vi "Autosort Populate Ring Control.vi"(8 "error in (no error)":errorcluster, 10 "Selected Index":i32, 11 "Ring Refnum":refnum<vi>) -> (0 "error out":errorcluster)   [LabVIEW 2016]
uses:
  Autosort Parameters Set.vi
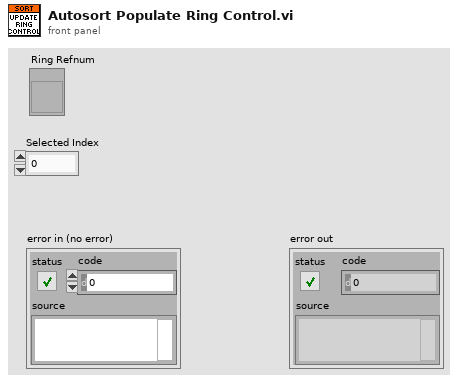
[diagram p1: front panel]
types:
  T1 = typedef "Autosort Parameters.ctl" = cluster{"Name":string, "Min Vel":dbl, "Trigger Ch":i32, "MaxVel":dbl, "Width":i32, "Pre Impuls":i32, "Post Impuls":i32, "Pitch":dbl, "Other Trigger":bool, "Cross Corr":bool}
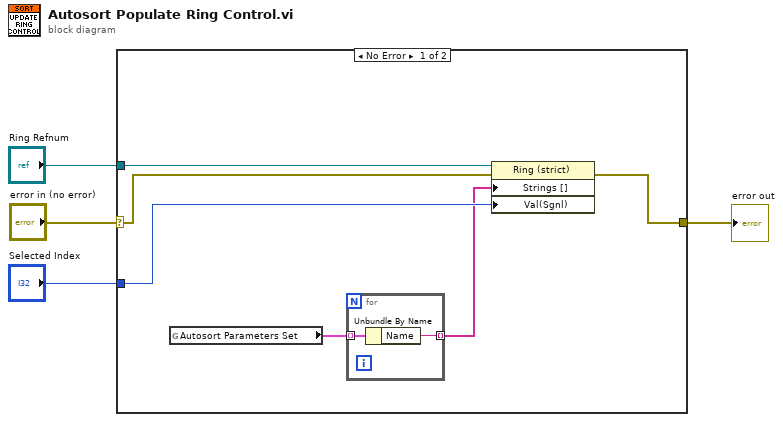
[diagram p0: block diagram]
diagram:
  n1 = case shown="No Error" "error in (no error)" {
    selector: "error in (no error)" -> [w9 w13]
    tunnel: "Ring Refnum" -> [w10 _]
    tunnel: "Selected Index" -> [w8 _]
    tunnel: [w7 w13] -> w1
    frame No Error {
      n2 = global read "Autosort Parameters Set.vi" "Autosort Parameters Set"() -> (w6:T1[])
      n3 = for {
        tunnel: w6 -> [w12] mode=indexing
        tunnel: [w11] -> w5 mode=indexing
        n4 = Unbundle By Name(w12) -> ("Name"=w11:string)
      }
      n5 = property on="Property Node" class="Ring (strict)"(reference=w10, error in=w9, "Strings []"=w5, "Val(Sgnl)"=w8) -> (error out=w7:errorcluster)  [unwired: 1 out]
    }
    frame Error {
    }
  }
  "error out" <- w1
